vi "Engine-SystemAI-Ch01.vi"(1 "dt [s]":sgl=1.0 format="%0.2f", 2 "AI01 [V]":sgl) -> (0 "AI01":T1)   [LabVIEW 2016, in "DSI-RT.lvlib"]
uses:
  DSI-RT.lvlib
  Shared/Typedefs/Engine-Channel.ctl
  <vilib>/Analysis/3filter.llb/Filter Passband Type.ctl
  <vilib>/addons/Software Calibration Management/xSCM/Controls/TBL1D.ctl
  <vilib>/addons/Software Calibration Management/xSCM/Controls/TLU1D.ctl
  <vilib>/addons/Software Calibration Management/xSCM/CalPoint.xnode
  <vilib>/ptbypt/NI_PtbyPt.lvlib
  <vilib>/Analysis/NI_AALBase.lvlib
  Shared/DSI-Shared.lvlib
  <vilib>/addons/Software Calibration Management/xSCM/ni_scm.dll
  <vilib>/addons/Software Calibration Management/xSCM/SCM-API.lvlib
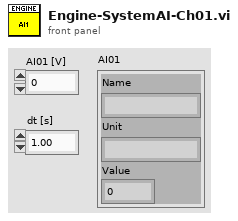
[diagram p1: front panel]
types:
  T1 = typedef "DSI-Shared.lvlib/Engine-Channel.ctl" = cluster{"Name":string, "Unit":string, "Value":sgl}
  T2 = typedef "NI_AALBase.lvlib/Filter Passband Type.ctl" = enum32{"Lowpass", "Highpass", "Bandpass", "Bandstop"}
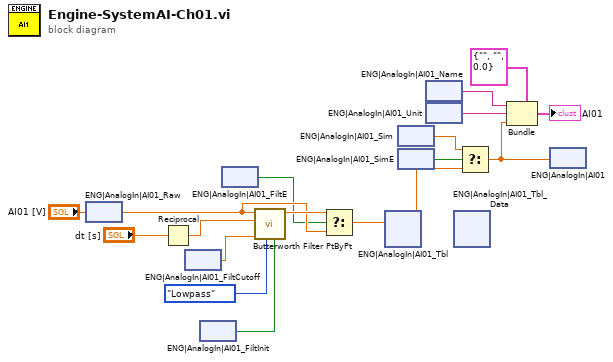
[diagram p0: block diagram]
diagram:
  n1 = xnode "ENG|AnalogIn|AI01_Raw"("Value"="AI01 [V]") -> ()
  n2 = Reciprocal(x="dt [s]") -> (1/x=w14:sgl)
  n3 = xnode "ENG|AnalogIn|AI01_FiltCutoff"() -> ("Value"=w1:sgl)
  n4 = xnode "ENG|AnalogIn|AI01_FiltInit"() -> ("Value"=w12:bool)
  n5 = xnode "ENG|AnalogIn|AI01_FiltE"() -> ("Value"=w2:bool)
  n6 = call <vilib>:"Butterworth Filter PtByPt.vi"("initialize"=w12, "filter type"=Filter_Passband_Type."Lowpass", "low cutoff freq: fl"=w1, "sampling freq: fs"=w14, "x"="AI01 [V]") -> ("Filtered x"=w11:dbl)  [unwired: 4 in, 1 out]
  n7 = Select(t=w11, s=w2, f="AI01 [V]") -> (s? t:f=w10:dbl)
  n8 = xnode "ENG|AnalogIn|AI01_Tbl"("X Index"=w10) -> ("Y"=w9:sgl)
  n9 = xnode "ENG|AnalogIn|AI01_Sim"() -> ("Value"=w16:sgl)
  n10 = xnode "ENG|AnalogIn|AI01_SimE"() -> ("Value"=w17:bool)
  n11 = xnode "ENG|AnalogIn|AI01_Name"() -> ("Value"=w7:string)
  n12 = xnode "ENG|AnalogIn|AI01_Unit"() -> ("Value"=w6:string)
  n13 = xnode "ENG|AnalogIn|AI01_Tbl_Data"() -> ()  [unwired: 1 out]
  n14 = Select(t=w16, s=w17, f=w9) -> (s? t:f=w4:sgl)
  n15 = Bundle(cluster=T1 {"Name"="", "Unit"="", "Value"=0.0} ("AI01"), "Name"=w7, "Unit"=w6, "Value"=w4) -> (→"AI01":T1)
  n16 = xnode "ENG|AnalogIn|AI01"("Value"=w4) -> ()
